vi "new sequence dialog.vi"(10 "Existing Sequences":string[](array[string]), 11 "Sequence Name":string) -> (2 "Canceled?":bool, 3 "Sequence Name Out":string)   [LabVIEW 2015, in "Simple Sequencer TBM editor node.lvclass"]
doc: "Displays a dialog that allows a user to enter the name of a new sequence."
uses:
  Simple Sequencer TBM editor node.lvclass
panel:
  in  "Cancel":bool
  in  "OK":bool
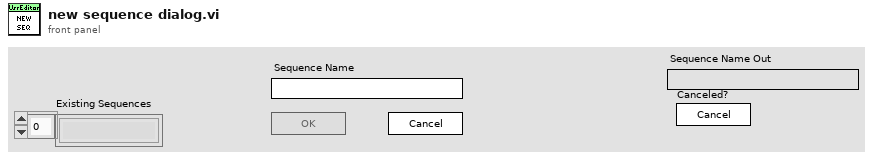
[diagram p1: front panel]
types:
  T1 = enum8{"Enabled", "Disabled", "Disabled and Grayed Out"}
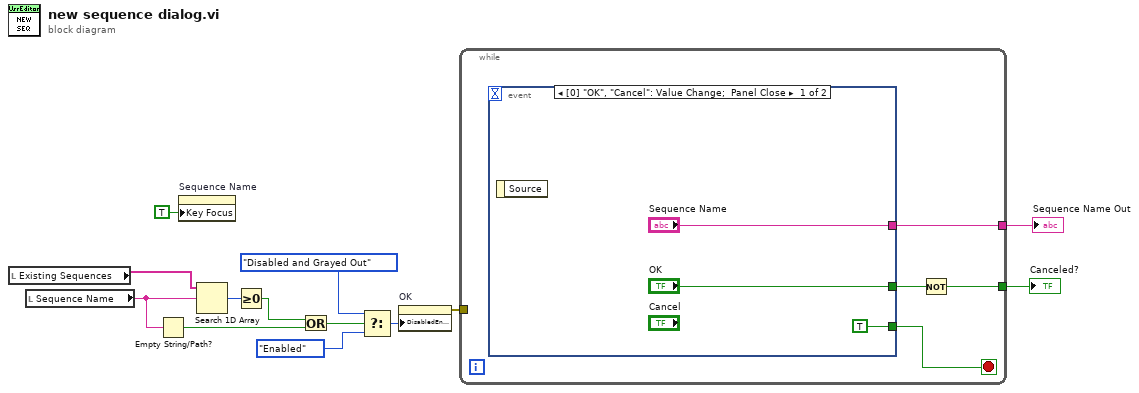
[diagram p0: block diagram]
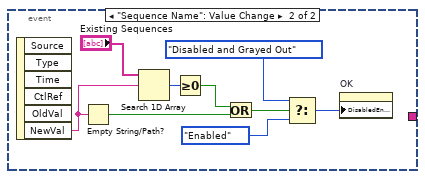
[diagram p2: hidden frame]
diagram:
  n1 = local read "Existing Sequences"() -> (w11:string[])
  n2 = local read "Sequence Name"() -> (w10:string)
  n3 = Empty String/Path?(string/path=w10) -> (empty?=w3:bool)
  n4 = property on="Sequence Name" class="Str"("Key Focus"=TRUE) -> ()  [unwired: 2 in, 2 out]
  n5 = Search 1D Array(1D array=w11, element=w10) -> (index of element=w12:i32)  [unwired: 1 in]
  n6 = Greater Or Equal To 0?(x=w12) -> (x >= 0?=w9:bool)
  n7 = Or(x=w9, y=w3) -> (x .or. y?=w8:bool)
  n8 = Select(t=T1."Disabled and Grayed Out" ("Disabled"), s=w8, f=T1."Enabled" ("Disabled")) -> (s? t:f=w7:T1)
  n9 = property on="OK" class="Bool"("DisabledEnum"=w7) -> (error out=w6:errorcluster)  [unwired: 2 in, 1 out]
  n10 = while {
    tunnel: [w17] -> w13
    tunnel: w6 -> [_]
    tunnel: [w14] -> w1
    stop <- w16 stop-if-true
    n11 = event shown="[0] \"OK\", \"Cancel\": Value Change;  Panel Close" {
      selector: _ -> [_ _]
      dyn-events: _ -> [_ _]
      timeout: _ -> [_ _]
      tunnel: ["OK" _] -> w15
      tunnel: ["Sequence Name" _] -> w17
      tunnel: [TRUE _] -> w16
      event "OK", "Cancel": Value Change; Panel Close {
        n12 = event-data() -> ()  [unwired: 1 in, 1 out]
      }
      event "Sequence Name": Value Change {
        n13 = event-data() -> ("NewVal"=w21:string)  [unwired: 1 in, 5 out]
        n14 = Empty String/Path?(string/path=w21) -> (empty?=w24:bool)
        n15 = Search 1D Array(1D array="Existing Sequences", element=w21) -> (index of element=w29:i32)  [unwired: 1 in]
        n16 = Greater Or Equal To 0?(x=w29) -> (x >= 0?=w28:bool)
        n17 = Or(x=w28, y=w24) -> (x .or. y?=w27:bool)
        n18 = Select(t=T1."Disabled and Grayed Out" ("Disabled"), s=w27, f=T1."Enabled" ("Disabled")) -> (s? t:f=w23:T1)
        n19 = property on="OK" class="Bool"("DisabledEnum"=w23) -> ()  [unwired: 2 in, 2 out]
      }
    }
    n20 = Not(x=w15) -> (.not. x?=w14:bool)
  }
  "Canceled?" <- w1
  "Sequence Name Out" <- w13
